vi "Acq Initiate.vi"(0 "session in":refnum<class "Digitizer Control.lvclass">, 1 "sample count (-1)":i64[](array[numeric]), 2 "record count (1)":i64[](array[numeric]), 3 "desired delay (s)":dbl, 4 "desired digital gain (dB)":dbl[](array[numeric]), 5 "error in (no error)":errorcluster, 7 "desired digital offset (V)":dbl[](array[numeric])) -> (13 "actual digital offset (V)":dbl[](array[numeric]), 14 "session out":refnum<class "Digitizer Control.lvclass">, 15 "actual sample count":i64[](array[numeric]), 16 "elements to read":i64[](array[numeric]), 17 "actual delay (s)":dbl, 18 "actual digital gain (dB)":dbl[](array[numeric]), 19 "error out":errorcluster)   [LabVIEW 2021, in "Digitizer Control.lvclass"]
doc: "Initiates a waveform acquisition. Use the <B>Acq Configure Channel.vi</B> to configure the channel parameters, the <B>Acq Configure Transfer.vi</B> to configure the waveform transfer, and the <B>Acq Configure Start Trigger.vi</B> to configure the start trigger before calling this VI. After the acquisition is initiated, use the <B>Acq Fetch Waveform.vi</B> to fetch the samples of the acquired waveform(s). Use the <B>Acq Get Status.vi</B> to check the acquisition status and the <B>Acq Stop.vi</B> to stop an acquisition.\n\nInputs:\n\n<B>session in</B>: The device session.\n\n<B>sample count</B>: The number of samples per record to acquire. Use a negative value to initiate an infinite acquisition. The default value of this parameter is -1. This input is an array, the n-th element corresponds to the n-th channel.\n\n<B>record count</B>: The number of records to acquire. Use a negative value to acquire an infinite number of records. The default value of this parameter is 1. This input is an array, the n-th element corresponds to the n-th channel.\n\n<B>desired delay (s)</B>: The desired DSP path delay. The minimum delay is returned on the <B>DSP delay (s)</B> output of the <B>Acq Configure Channel.vi</B>, smaller values are coerced to this minimum delay. Use this input to apply additional delay to the beginning of the acquisition.\n\n<B>desired digital gain (dB)</B>: The desired digital gain, given in decibels. This input is an array, the n-th element corresponds to the n-th channel.\n\n<B>desired digital offset (V)</B>: The desired digital offset to apply on the DSP input, given in Volts. This input is an array, the n-th element corresponds to the n-th channel.\n\nOutputs:\n\n<B>session out</B>: The device session passed on the <B>session in</B> input.\n\n<B>actual sample count</B>: The actual number of samples per record to acquire in case of a finite acquisition. In case of an infinite acquisition this output returns -1. This output is an array, the n-th element corresponds to the n-th channel.\n\n<B>elements to read</B>: The number of elements to read from the host DMA buffer to fetch an acquired waveform (a single record) in case of a finite acquisition. In case of an infinite acquisition this output returns -1. This output is an array, the n-th element corresponds to the n-th channel.\n\n<B>actual delay (s)</B>: The actual DSP path delay.\n\n<B>actual digital gain (dB)</B>: The actual digital gain, given in decibels. This output is an array, the n-th element corresponds to the n-th channel.\n\n<B>actual digital offset (V)</B>: The actual digital offset applied on the DSP input, given in Volts. This output is an array, the n-th element corresponds to the n-th channel."
uses:
  Digitizer Control.lvclass
  Digitizer Control.lvclass/Digitizer Control.ctl
  <vilib>/Utility/error.llb/Error Cluster From Error Code.vi
  <vilib>/rvi/errors/niLvFpgaAdjustHostInterfaceError.vi
  <instrlib>/_niInstr/Streaming/v1/Host/Public/Start Finite Stream.vi
  <instrlib>/_niInstr/Streaming/v1/Host/Public/Start Continuous Stream.vi
  <vilib>/ErrorRing/Error Ring.xnode
  <vilib>/rvi/interface/nirviReadWriteControl/nirviReadWriteControl.xnode
  <instrlib>/_niInstr/Streaming/v1/Host/niInstr Streaming v1 Host.lvlib
  NiFpgaLv.dll
  <vilib>/rvi/interface/Simulation/niFpgaSimulationCallBeginRW.vi
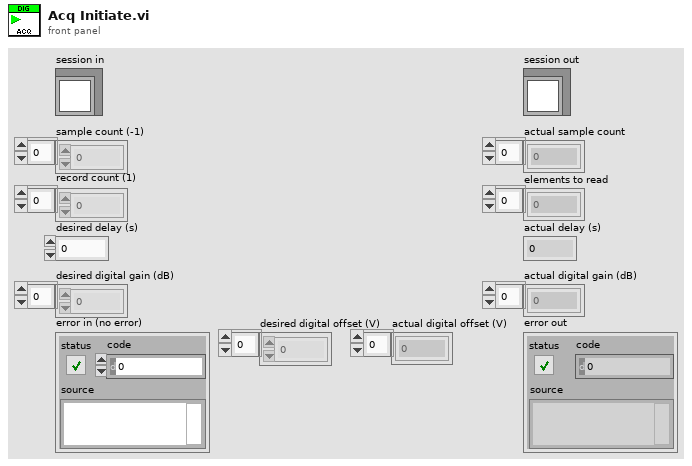
[diagram p1: front panel]
types:
  T1 = typedef "Digitizer Control.lvclass/Acq Session Data.ctl" = cluster{"ADC sampling rate":dbl, "SCTL rate":dbl, "DMA element size (bits)":i32, "sample size (bits)":i32[], "DMA/memory interface width (DMA elements)":i32, "transfer size (bits)":i32[], "stream instance":i32[], "trigger instance":u32, "group delay (s)":dbl, "data delay (s)":dbl, "target delay (s)":dbl, "trigger tracking enabled":bool, "channel configured":bool, "enabled channels":bool[], "transfer configured":bool, "dsp bypass":bool, "fractional decimator input rate":dbl, "fractional decimator output rate":dbl, "sample scale factor":dbl[], "memory size":u64[], "FIFO size":u64}
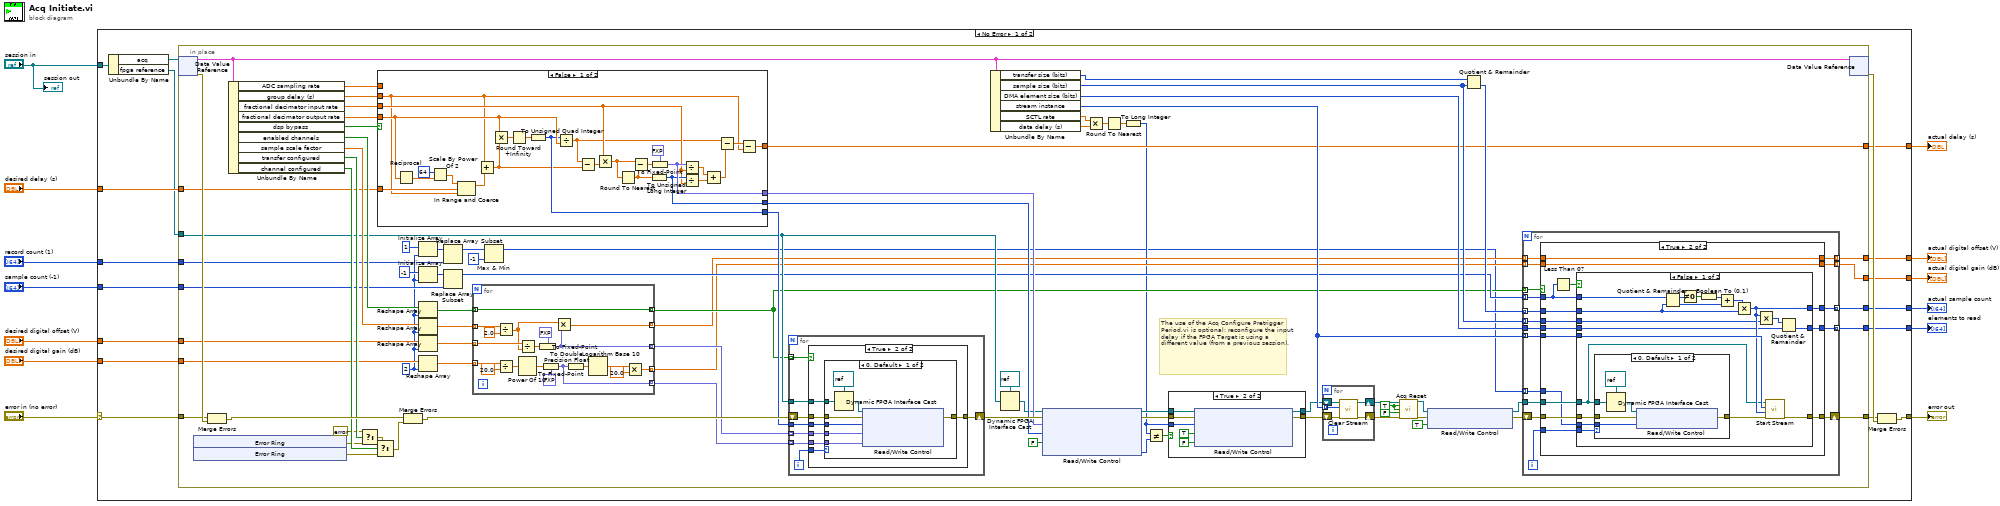
[diagram p0: block diagram]
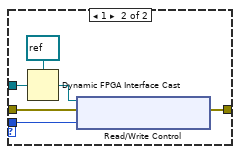
[diagram p4: hidden frame]
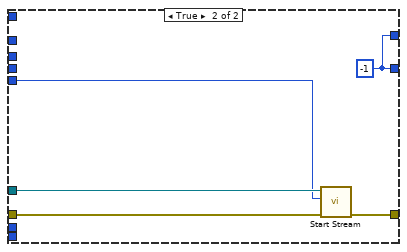
[diagram p5: hidden frame]
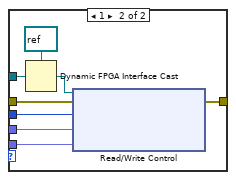
[diagram p7: hidden frame]
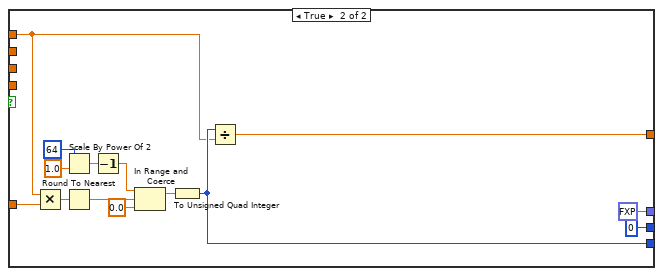
[diagram p8: hidden frame]
diagram:
  n1 = case shown="No Error" "error in (no error)" {
    selector: "error in (no error)" -> [w28 w295]
    tunnel: [w25 w295] -> w12
    tunnel: "sample count (-1)" -> [w27 _]
    tunnel: [w29 _] -> w10
    tunnel: "session in" -> [w17 _]
    tunnel: "desired delay (s)" -> [w24 _]
    tunnel: [w23 _] -> w8
    tunnel: "desired digital offset (V)" -> [w22 _]
    tunnel: [w21 _] -> w6
    tunnel: "desired digital gain (dB)" -> [w20 _]
    tunnel: [w19 _] -> w4
    tunnel: [w18 _] -> w3
    tunnel: "record count (1)" -> [w14 _]
    frame No Error {
      n2 = Unbundle By Name(w17) -> ("acq"=w16:refnum<data-value>, "fpga reference"=w15:refnum<k20>)
      n3 = in-place {
        in-place-border: [w77] -> w26
        in-place-border: [w100] -> w29
        in-place-border: w28 -> [w98]
        in-place-border: w27 -> [w67]
        in-place-border: w24 -> [w94]
        in-place-border: [w73] -> w23
        in-place-border: w22 -> [w65]
        in-place-border: [w50] -> w21
        in-place-border: w20 -> [w63]
        in-place-border: [w49] -> w19
        in-place-border: [w86] -> w18
        in-place-border: w15 -> [w56]
        in-place-border: w14 -> [w45]
        w46 = 2 ("dimension size")
        w96 = TRUE ("reset dsp")
        # "The use of the Acq Configure Pretrigger Period.vi is optional: reconfigure the input delay if the FPGA Target is using a different value (from a previous session)."
        n4 = in-place-dvr #1(w16) -> (w72:T1, w101:errorcluster)
        n5 = xnode "Error Ring"() -> ("error out"=w103:errorcluster)
        n6 = xnode "Error Ring"() -> ("error out"=w104:errorcluster)
        n7 = Merge Errors(w98, w101) -> (w109:errorcluster)
        n8 = Unbundle By Name(w72) -> ("ADC sampling rate"=w71:dbl, "group delay (s)"=w74:dbl, "fractional decimator input rate"=w90:dbl, "fractional decimator output rate"=w93:dbl, "dsp bypass"=w70:bool, "enabled channels"=w108:bool[], "sample scale factor"=w107:dbl[], "transfer configured"=w106:bool, "channel configured"=w105:bool)
        n9 = Select(t=errorcluster {"status"=FALSE, "code"=0, "source"=""}, s=w106, f=w103) -> (s? t:f=w76:errorcluster)
        n10 = Select(t=w76, s=w105, f=w104) -> (s? t:f=w75:errorcluster)
        n11 = case shown="False" w70 {
          tunnel: w94 -> [w267 w284]
          tunnel: w93 -> [w264 _]
          tunnel: [w258 fxp<+/-,16,0> 0.0 ("acq.dsp.delay")] -> w92
          tunnel: [w257 u32 0] -> w91
          tunnel: w90 -> [w256 _]
          tunnel: [w252 w275] -> w58
          tunnel: w74 -> [w247 _]
          tunnel: [w246 w273] -> w73
          tunnel: w71 -> [_ w274]
          frame False {
            n12 = Reciprocal(x=w264) -> (1/x=w270:dbl)
            n13 = Scale By Power Of 2(n=i16 64, x=w270) -> (x*2^n=w268:dbl)
            n14 = In Range and Coerce(upper limit=w268, x=w267, lower limit=w247) -> (coerced(x)=w263:dbl)  [unwired: 1 out]
            n15 = Add(x=w247, y=w263) -> (x+y=w248:dbl)
            n16 = Multiply(x=w264, y=w248) -> (x*y=w266:dbl)
            n17 = Round Toward +Infinity(x=w266) -> (ceil(x): smallest int >= x=w265:dbl)
            n18 = To Unsigned Quad Integer(1:w265) -> (0:w252:u64)
            n19 = Divide(x=w252, y=w264) -> (x/y=w251:dbl)
            n20 = Subtract(x=w251, y=w248) -> (x-y=w262:dbl)
            n21 = Multiply(x=w256, y=w262) -> (x*y=w249:dbl)
            n22 = Round To Nearest(number=w249) -> (nearest integer value=w261:dbl)
            n23 = Subtract(x=w249, y=w261) -> (x-y=w260:dbl)
            n24 = To Unsigned Long Integer(number=w261) -> (unsigned 32bit integer=w257:u32)
            n25 = To Fixed-Point(fixed-point type=fxp<+/-,16,0> 0.0 ("acq.dsp.delay"), number=w260) -> (fixed-point=w258:fxp<+/-,16,0>)
            n26 = Divide(x=w258, y=w256) -> (x/y=w250:dbl)
            n27 = Divide(x=w257, y=w256) -> (x/y=w255:dbl)
            n28 = Add(x=w250, y=w255) -> (x+y=w254:dbl)
            n29 = Subtract(x=w251, y=w254) -> (x-y=w253:dbl)
            n30 = Subtract(x=w253, y=w247) -> (x-y=w246:dbl)
          }
          frame True {
            n31 = Multiply(x=w274, y=w284) -> (x*y=w283:dbl)
            n32 = Scale By Power Of 2(n=i16 64, x=1.0) -> (x*2^n=w278:dbl)
            n33 = Round To Nearest(number=w283) -> (nearest integer value=w282:dbl)
            n34 = Decrement(x=w278) -> (x-1=w277:dbl)
            n35 = In Range and Coerce(upper limit=w277, x=w282, lower limit=0.0 ("x")) -> (coerced(x)=w276:dbl)  [unwired: 1 out]
            n36 = To Unsigned Quad Integer(1:w276) -> (0:w275:u64)
            n37 = Divide(x=w275, y=w274) -> (x/y=w273:dbl)
          }
        }
        n38 = Merge Errors(w109, w75) -> (w110:errorcluster)
        n39 = Initialize Array(i64 1 ("element"), w46) -> (w48:i64[])
        n40 = Initialize Array(i64 -1 ("element"), w46) -> (w68:i64[])
        n41 = Reshape Array(w108, w46) -> (w62:bool[])
        n42 = Reshape Array(w107, w46) -> (w66:dbl[])
        n43 = Reshape Array(w65, w46) -> (w64:dbl[])
        n44 = Reshape Array(w63, w46) -> (w61:dbl[])
        n45 = Replace Array Subset(array=w48, new element=w45) -> (w32:i64[])  [unwired: 1 in]
        n46 = Replace Array Subset(array=w68, new element=w67) -> (w54:i64[])  [unwired: 1 in]
        n47 = for {
          tunnel: w66 -> [w229] mode=indexing
          tunnel: w64 -> [w245] mode=indexing
          tunnel: w62 -> [w235] mode=indexing
          tunnel: w61 -> [w237] mode=indexing
          tunnel: [w242] -> w59 mode=indexing
          tunnel: [w241] -> w52 mode=indexing
          tunnel: [w235] -> w53 mode=indexing
          tunnel: [w231] -> w60 mode=indexing
          tunnel: [w230] -> w51 mode=indexing
          n48 = Divide(x=w229, y=2.0) -> (x/y=w227:dbl)
          n49 = Divide(x=w237, y=20.0) -> (x/y=w239:dbl)
          n50 = Power Of 10(x=w239) -> (10^x=w240:dbl)
          n51 = Divide(x=w245, y=w227) -> (x/y=w243:dbl)
          n52 = To Fixed-Point(fixed-point type=fxp<+/-,18,1> 0.0, number=w243) -> (fixed-point=w242:fxp<+/-,18,1>)
          n53 = To Fixed-Point(fixed-point type=fxp<+/-,24,3> 0.0 ("gain I"), number=w240) -> (fixed-point=w231:fxp<+/-,24,3>)
          n54 = Multiply(x=w227, y=w242) -> (x*y=w241:dbl)
          n55 = To Double Precision Float(number=w231) -> (double precision float=w232:dbl)
          n56 = Logarithm Base 10(1:w232) -> (0:w233:dbl)
          n57 = Multiply(x=w233, y=20.0) -> (x*y=w230:dbl)
        }
        n58 = Max & Min(x=w32, y=i64 -1) -> (max(x,y)=w31:i64[])  [unwired: 1 out]
        n59 = for {
          tunnel: w56 -> [w201]
          tunnel: w60 -> [w200] mode=indexing
          tunnel: w59 -> [w199] mode=indexing
          tunnel: w58 -> [w198]
          tunnel: w53 -> [w197] mode=indexing
          shift-right: [w195] -> w111
          shift-left: w110 -> [w202]
          i -> [w196]
          n60 = case shown="True" w197 {
            tunnel: w196 -> [_ w210]
            tunnel: w202 -> [w203 w209]
            tunnel: w201 -> [_ w208]
            tunnel: w200 -> [_ w207]
            tunnel: w199 -> [_ w206]
            tunnel: w198 -> [_ w205]
            tunnel: [w203 w204] -> w195
            frame False {
            }
            frame True {
              n61 = case shown="0, Default" w210 {
                tunnel: w209 -> [w216 w224]
                tunnel: w208 -> [w217 w225]
                tunnel: [w214 w222] -> w204
                tunnel: w207 -> [w213 w221]
                tunnel: w206 -> [w212 w220]
                tunnel: w205 -> [w211 w219]
                frame 0, Default {
                  n62 = Dynamic FPGA Interface Cast(Session In=refnum<k20> refnum ("FPGA Interface"), Type=w217) -> (Session Out=w215:refnum<k20>)
                  n63 = xnode "Read/Write Control"("FPGA VI Reference In"=w215, "error in"=w216, "stream.initial ignore 0"=w211, "acq.dsp.offset 0"=w212, "acq.dsp.gain 0"=w213) -> ("error out"=w214:errorcluster)  [unwired: 1 out]
                }
                frame 1 {
                  n64 = Dynamic FPGA Interface Cast(Session In=refnum<k20> refnum ("FPGA Interface"), Type=w225) -> (Session Out=w223:refnum<k20>)
                  n65 = xnode "Read/Write Control"("FPGA VI Reference In"=w223, "error in"=w224, "stream.initial ignore 1"=w219, "acq.dsp.offset 1"=w220, "acq.dsp.gain 1"=w221) -> ("error out"=w222:errorcluster)  [unwired: 1 out]
                }
              }
            }
          }
        }
        n66 = Unbundle By Name(w72) -> ("transfer size (bits)"=w82:i32[], "sample size (bits)"=w85:i32[], "DMA element size (bits)"=w83:i32, "stream instance"=w84:i32[], "SCTL rate"=w41:dbl, "data delay (s)"=w42:dbl)
        n67 = Dynamic FPGA Interface Cast(Session In=refnum<k20> refnum ("FPGA Interface"), Type=w56) -> (Session Out=w55:refnum<k20>)
        n68 = xnode "Read/Write Control"("FPGA VI Reference In"=w55, "error in"=w111, "acq.dsp.delay"=w92, "acq.dsp.integer delay"=w91, "acq.stream.start enable"=FALSE) -> ("FPGA VI Reference Out"=w39:refnum<k20>, "error out"=w40:errorcluster, "flexrio.buffer.delay.clocks 0"=w35:u16)
        n69 = Multiply(x=w41, y=w42) -> (x*y=w44:dbl)
        n70 = Round To Nearest(number=w44) -> (nearest integer value=w43:dbl)
        n71 = To Long Integer(number=w43) -> (32bit integer=w36:i32)
        n72 = Not Equal?(x=w36, y=w35) -> (x != y?=w34:bool)
        n73 = case shown="True" w34 {
          tunnel: w40 -> [w113 w120]
          tunnel: w39 -> [w112 w119]
          tunnel: w36 -> [_ w118]
          tunnel: [w113 w115] -> w38
          tunnel: [w112 w114] -> w37
          frame False {
          }
          frame True {
            n74 = xnode "Read/Write Control"("FPGA VI Reference In"=w119, "error in"=w120, "flexrio.buffer.delay.clocks 0"=w118, "flexrio.buffer.delay.reset 0"=TRUE, "flexrio.buffer.delay.reset 0"=FALSE) -> ("FPGA VI Reference Out"=w114:refnum<k20>, "error out"=w115:errorcluster)
          }
        }
        n75 = for {
          tunnel: w84 -> [w191] mode=indexing
          shift-right: [w194] -> w99
          shift-left: w38 -> [w192]
          shift-right: [w193] -> w97
          shift-left: w37 -> [w190]
          n76 = call <instrlib>:"Clear Stream.vi"("error in (no error)"=w192, "stream index"=w191, "refnum in"=w190) -> ("error out"=w194:errorcluster, "refnum out"=w193:refnum<k20>)  [unwired: 7 in]
        }
        n77 = call "Acq Reset.vi"("fpga reference in"=w97, "reset dsp"=w96, "reset stream control"=w96, "reset waveform streaming"=FALSE ("reset host streaming"), "error in (no error)"=w99) -> ("fpga reference out"=w80:refnum<k20>, "error out"=w81:errorcluster)  [unwired: 9 in]
        n78 = xnode "Read/Write Control"("FPGA VI Reference In"=w80, "error in"=w81, "acq.stream.start enable"=TRUE) -> ("FPGA VI Reference Out"=w78:refnum<k20>, "error out"=w79:errorcluster)
        n79 = Quotient & Remainder(x=w82, y=w85) -> (floor(x/y)=w87:i32[])  [unwired: 1 out]
        n80 = for {
          tunnel: [w137] -> w100 mode=indexing
          tunnel: w87 -> [w136] mode=indexing
          tunnel: [w135] -> w86 mode=indexing
          tunnel: w85 -> [w134] mode=indexing
          tunnel: w84 -> [w133] mode=indexing
          tunnel: w83 -> [w132]
          tunnel: w78 -> [w130]
          tunnel: w54 -> [w128] mode=indexing
          shift-right: [w129] -> w77
          shift-left: w79 -> [w131]
          tunnel: w53 -> [w127] mode=indexing
          tunnel: w52 -> [w126] mode=indexing
          tunnel: w51 -> [w125] mode=indexing
          tunnel: [w124] -> w50 mode=indexing
          tunnel: [w123] -> w49 mode=indexing
          tunnel: w31 -> [w122] mode=indexing
          i -> [w121]
          n81 = case shown="True" w127 {
            tunnel: [_ w153] -> w137
            tunnel: w136 -> [_ w151]
            tunnel: [_ w150] -> w135
            tunnel: w134 -> [_ w149]
            tunnel: w133 -> [_ w148]
            tunnel: w132 -> [_ w147]
            tunnel: w131 -> [w138 w146]
            tunnel: w130 -> [_ w145]
            tunnel: [w138 w144] -> w129
            tunnel: w128 -> [_ w143]
            tunnel: w126 -> [_ w142]
            tunnel: w125 -> [_ w141]
            tunnel: [_ w142] -> w124
            tunnel: [_ w141] -> w123
            tunnel: w122 -> [_ w140]
            tunnel: w121 -> [_ w139]
            frame False {
            }
            frame True {
              n82 = Less Than 0?(x=w143) -> (x < 0?=w152:bool)
              n83 = case shown="False" w152 {
                tunnel: w148 -> [w172 w186]
                tunnel: [w159 w185] -> w153
                tunnel: w143 -> [w170 _]
                tunnel: w145 -> [w157 w187]
                tunnel: w146 -> [w156 w189]
                tunnel: [w171 w188] -> w144
                tunnel: w151 -> [w164 _]
                tunnel: [w163 w185] -> w150
                tunnel: w149 -> [w162 _]
                tunnel: w147 -> [w160 _]
                tunnel: w140 -> [w154 _]
                tunnel: w139 -> [w158 _]
                frame False {
                  n84 = case shown="0, Default" w158 {
                    tunnel: w157 -> [w177 w183]
                    tunnel: w156 -> [w175 w181]
                    tunnel: [w174 w180] -> w155
                    tunnel: w154 -> [w173 w179]
                    frame 0, Default {
                      n85 = Dynamic FPGA Interface Cast(Session In=refnum<k20> refnum ("FPGA Interface"), Type=w177) -> (Session Out=w176:refnum<k20>)
                      n86 = xnode "Read/Write Control"("FPGA VI Reference In"=w176, "error in"=w175, "stream.num records 0"=w173) -> ("error out"=w174:errorcluster)  [unwired: 1 out]
                    }
                    frame 1 {
                      n87 = Dynamic FPGA Interface Cast(Session In=refnum<k20> refnum ("FPGA Interface"), Type=w183) -> (Session Out=w182:refnum<k20>)
                      n88 = xnode "Read/Write Control"("FPGA VI Reference In"=w182, "error in"=w181, "stream.num records 1"=w179) -> ("error out"=w180:errorcluster)  [unwired: 1 out]
                    }
                  }
                  n89 = Quotient & Remainder(x=w170, y=w164) -> (x-y*floor(x/y)=w169:i64, floor(x/y)=w166:i64)
                  n90 = Not Equal To 0?(x=w169) -> (x != 0?=w168:bool)
                  n91 = Boolean To (0,1)(Boolean=w168) -> (0, 1=w167:i16)
                  n92 = Add(x=w167, y=w166) -> (x+y=w165:i64)
                  n93 = Multiply(x=w165, y=w164) -> (x*y=w163:i64)
                  n94 = Multiply(x=w163, y=w162) -> (x*y=w161:i64)
                  n95 = call-poly <instrlib>:"Start Stream.vi"("error in (no error)"=w155, "num samples"=w163, "stream index"=w172, "refnum in"=w157) -> ("error out"=w171:errorcluster)  [unwired: 6 in, 1 out]
                  n96 = Quotient & Remainder(x=w161, y=w160) -> (floor(x/y)=w159:i64)  [unwired: 1 out]
                }
                frame True {
                  w185 = i64 -1
                  n97 = call-poly <instrlib>:"Start Stream.vi"("error in (no error)"=w189, "stream index"=w186, "refnum in"=w187) -> ("error out"=w188:errorcluster)  [unwired: 7 in, 1 out]
                }
              }
            }
          }
        }
        n98 = in-place-dvr #1(w72) -> (w30:errorcluster)  [unwired: 1 out]
      }
      n99 = Merge Errors(w26, w30) -> (w25:errorcluster)
    }
    frame Error {
    }
  }
  "error out" <- w12
  "elements to read" <- w10
  "actual digital offset (V)" <- w6
  "actual digital gain (dB)" <- w4
  "actual delay (s)" <- w8
  "actual sample count" <- w3
  "session out" <- "session in"
